vi "SPI Flash Write.vi"(6 "WriteLen":i32, 7 "pWriteData":u8, 9 "StartAddr":i32, 10 "SPIIndex":i32, 11 "DevHandle":i32) -> (3 "function return":i32, 5 "pWriteData out":u8)   [LabVIEW 2010, in "usb2spi.lvlib"]
doc: "int WINAPI SPI_FlashWrite(int DevHandle,int SPIIndex,int StartAddr,unsigned char *pWriteData,int WriteLen);"
uses:
  usb2spi.lvlib
  USB2XXX.dll
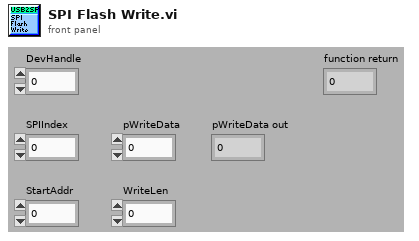
[diagram p1: front panel]
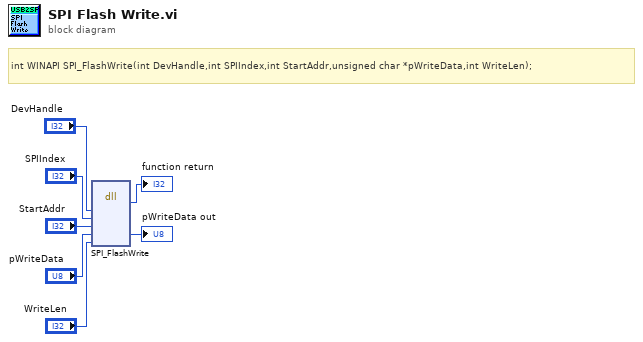
[diagram p0: block diagram]
diagram:
  # "int WINAPI SPI_FlashWrite(int DevHandle,int SPIIndex,int StartAddr,unsigned char *pWriteData,int WriteLen);"
  n1 = dll-call lib="G:/OtherWork/USB2XXX_Example/trunk/Labview/PublicFiles/usb2spi/USB2XXX.*" fn="SPI_FlashWrite"("DevHandle"="DevHandle", "SPIIndex"="SPIIndex", "StartAddr"="StartAddr", "pWriteData"="pWriteData", "WriteLen"="WriteLen") -> (→"function return":i32, "pWriteData"=→"pWriteData out":u8)  [unwired: 7 in, 2 out]
